vi "CTRnode.vi"(8 "error in":errorcluster) -> (0 "error out":errorcluster)   [LabVIEW 2024]
uses:
  Control/StreamCluster_TypeDef.ctl
  Control/streamIO_states.ctl
  <vilib>/Platform/TimedLoop/XDataNode/timing_clust.ctl
  <vilib>/Platform/TimedLoop/XDataNode/nitl_modes.ctl
  <vilib>/Platform/TimedLoop/XDataNode/wakeup.ctl
  Support/GlobalVars/StreamCluster.vi
  <vilib>/Platform/TimedLoop/TimeConversion.llb/rt-milliseconds-to-rel-time.vi
  <vilib>/Platform/TimedLoop/TimeConversion.llb/rt-milliseconds-to-timestamp.vi
  <vilib>/platform/TimedLoop/XDataNode/XDataNode.xnode
  <vilib>/Platform/TimedLoop/XDataNode/XDNodeRunTimeDep.lvlib
panel:
  out "element":dbl[][][](array[numeric])
  out "Manage Clock (ms)":cluster{"Period":i64, i64}(graph)
  out "Logging Clock (ms)":cluster{"Period":i64, i64}(graph)
  in  "stop":bool
  out "Streaming Clock (ms)":cluster{dbl, "Period":dbl}(graph)
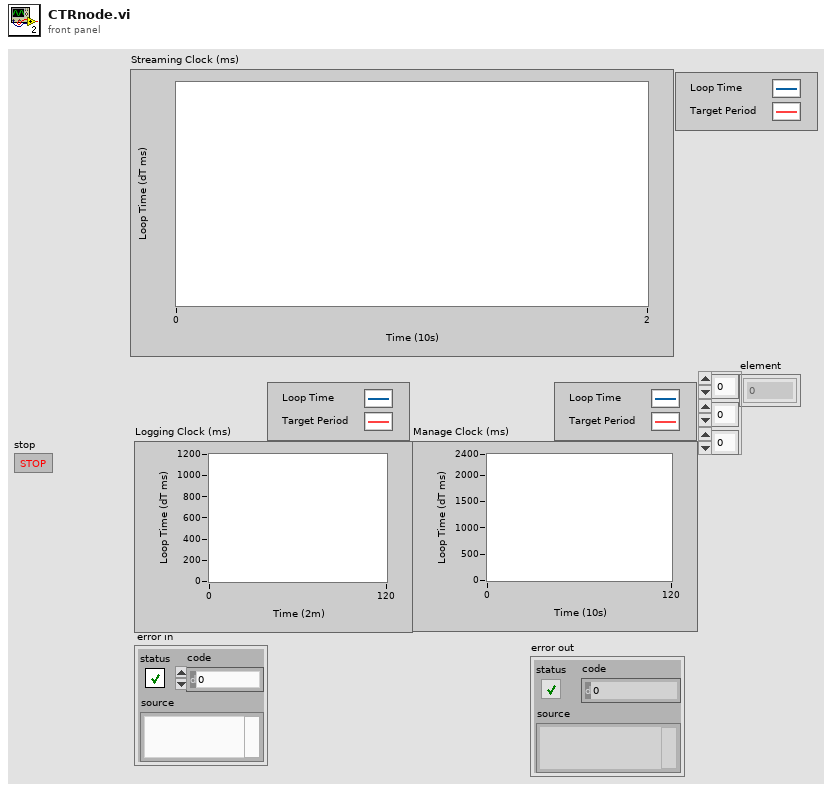
[diagram p1: front panel]
types:
  T1 = typedef "StreamCluster_TypeDef.ctl" = cluster{cluster{"stream state":T2, "TCP Remote Address":string, "TCP Connection ID":refnum<k5>, "DAQ Node":string, "DAQ Node ID":i32, "Writer Endpoint":refnum<k21>, "Reader Endpoint":refnum<k21>}[]}
  T2 = typedef "streamIO_states.ctl" = enum16{"Fault", "Initilize", "Stream", "Close"}
  T3 = typedef "XDNodeRunTimeDep.lvlib/timing_clust.ctl" = cluster{"Expected End [f-1]":u64, "Actual End [f-1]":u64, "Finished Late? [f-1]":bool, "Expected End [i-1]":u64, "Actual End [i-1]":u64, "Finished Late? [i-1]":bool, "Expected Start [i]":u64, "Actual Start [i]":u64, "Expected Start [f]":u64, "Actual Start [f]":u64, "Source Name":string, "Structure Name":string, "Period":i64, "Deadline":i64, "Offset":i64, "Start":i64, "Priority":i32, "Timeout":i32, "Mode":T4, "Wakeup Reason":T5, "Error":errorcluster, "Source Type":string, "Secondary Source Type":string, "Global End Time":u64, "Global Start Time":u64, "Frame Duration":u64, "Iteration Duration":u64, "Assigned CPU":i32, "I/O Scan Engine Mode":u32}
  T4 = typedef "XDNodeRunTimeDep.lvlib/nitl_modes.ctl" = enum32{"No Change", "Process missed periods, maintain original phase", "Discard missed periods, maintain original phase", "Process missed periods, ignore original phase", "Discard missed periods, ignore original phase"}
  T5 = typedef "XDNodeRunTimeDep.lvlib/wakeup.ctl" = enum32{"Normal", "Aborted", "Asynchronous wakeup", "Timing source error", "Timed loop error", "Timeout"}
  T6 = cluster{"stream state":T2, "TCP Remote Address":string, "TCP Connection ID":refnum<k5>, "DAQ Node":string, "DAQ Node ID":i32, "Writer Endpoint":refnum<k21>, "Reader Endpoint":refnum<k21>}[]
  T7 = cluster{"stream state":bool, "TCP Remote Address":bool, "TCP Connection ID":bool, "DAQ Node":bool, "DAQ Node ID":bool, "Writer Endpoint":bool, "Reader Endpoint":bool}
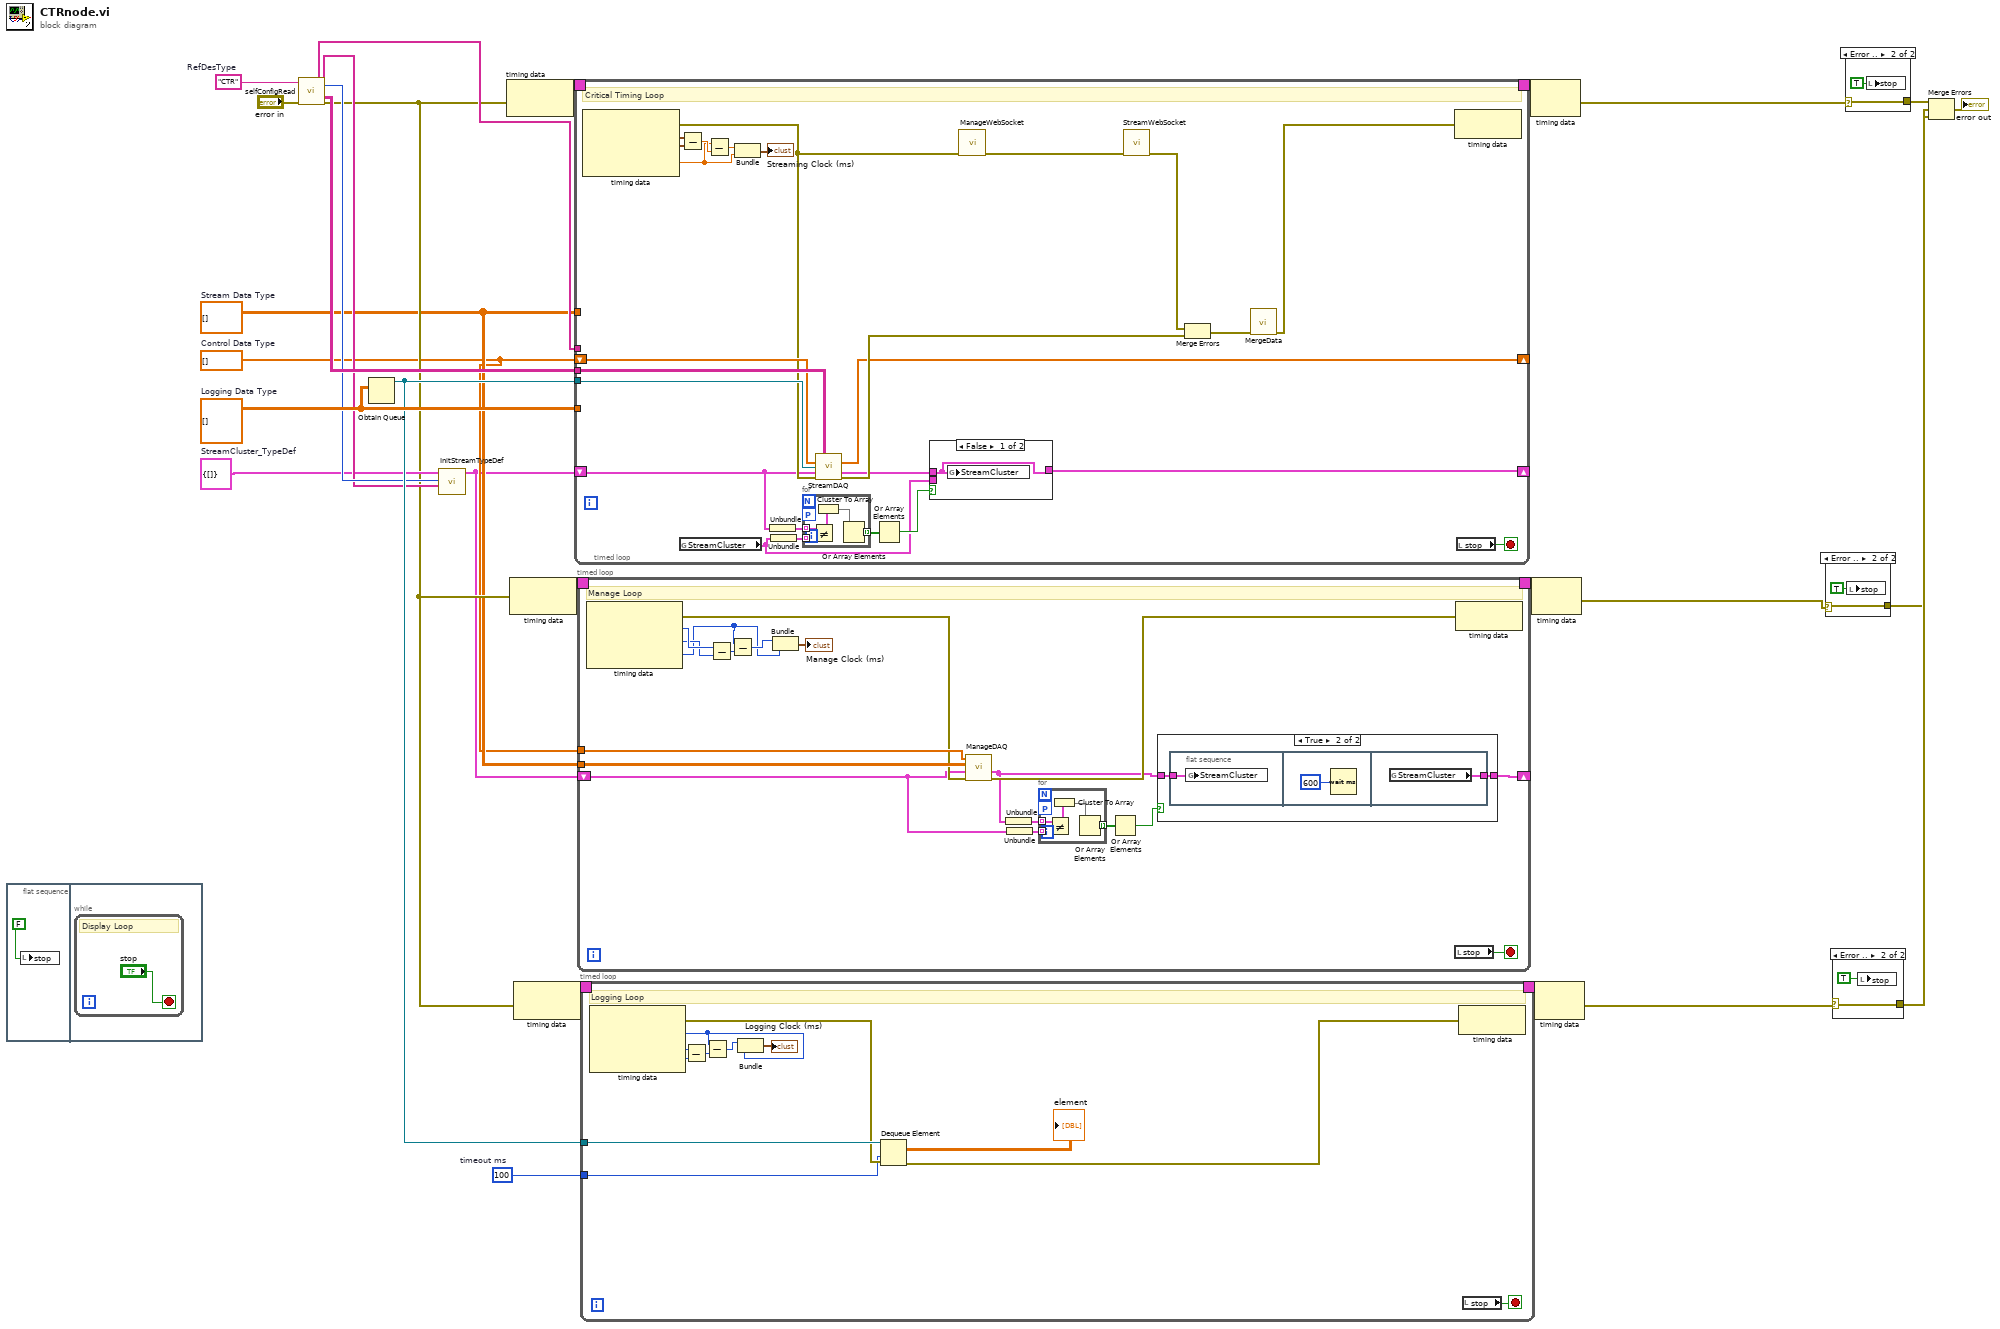
[diagram p0: block diagram]
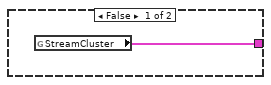
[diagram p3: hidden frame]
diagram:
  w9 = 100  # timeout ms
  w14 = T1 {[]}  # StreamCluster_TypeDef
  w4 = dbl[] []  # Control Data Type
  w20 = dbl[][][] []  # Logging Data Type
  w26 = "CTR"  # RefDesType
  w5 = dbl[][] []  # Stream Data Type
  n1 = flat-sequence {
    frame #0 {
      n2 = local write "stop"(FALSE ("stop")) -> ()
    }
    frame #1 {
      n3 = while {
        stop <- "stop" stop-if-true
        # "Display Loop"
      }
    }
  }
  n4 = call "selfConfigRead.vi"("RefDesType"=w26, "error in"="error in") -> ("Control refDes concat"=w19:string[], "DAQ Node Array"=w15:string[], "DAQ Node Count"=w16:i32, "Control refDes array"=w18:string[][], "error out"=w6:errorcluster)  [unwired: 11 in, 2 out]
  n5 = Obtain Queue(element data type=w20) -> (queue out=w17:refnum<queue>)  [unwired: 4 in, 2 out]
  n6 = call "InitStreamTypeDef.vi"("DAQ Node Array"=w15, "DAQ Node Count"=w16, "StreamCluster_TypeDef"=w14) -> ("StreamCluster_TypeDef"=w3:T1)  [unwired: 8 in]
  n7 = node-c288(w6) -> (w25:T3)
  n8 = node-c288(w6) -> (w8:T3)
  n9 = node-c288(w6) -> (w23:T3)
  n10 = timed-loop {
    timing: w25 -> [_]
    timing-out: [_] -> w24
    shift-right: [w30] -> _
    shift-left: w3 -> [w34]
    tunnel: w5 -> [_]
    tunnel: w20 -> [_]
    tunnel: w17 -> [w43]
    tunnel: w19 -> [_]
    tunnel: w18 -> [w42]
    shift-right: [w40] -> _
    shift-left: w4 -> [w39]
    stop <- w44 stop-if-true
    # "Critical Timing Loop"
    n11 = node-c288() -> (w38:errorcluster, w50:timestamp, w49:timestamp, w46:dbl)  [unwired: 1 in]
    n12 = global read "StreamCluster.vi" "StreamCluster"() -> (w31:T1)
    n13 = Subtract(x=w50, y=w49) -> (x-y=w48:dbl)
    n14 = Subtract(x=w46, y=w48) -> (x-y=w47:dbl)
    n15 = Bundle(w47, "Period"=w46) -> (→"Streaming Clock (ms)":cluster{dbl, "Period":dbl})  [unwired: 1 in]
    n16 = Unbundle(w34) -> (w37:T6)
    n17 = Unbundle(w31) -> (w36:T6)
    n18 = for {
      workers-P: _ -> [_]
      tunnel: w37 -> [w59] mode=indexing
      tunnel: w36 -> [w58] mode=indexing
      tunnel: [w55] -> w35 mode=indexing
      n19 = Not Equal?(x=w59, y=w58) -> (x != y?=w57:T7)
      n20 = Cluster To Array(cluster=w57) -> (array=w56:bool[])
      n21 = Or Array Elements(Boolean array=w56) -> (logical OR=w55:bool)
    }
    n22 = call "StreamDAQ.vi"("Control refDes array"=w42, "Control Data Type"=w39, "Logging Queue"=w43, "StreamCluster_TypeDef"=w34, "error in"=w38) -> ("Control Data Out"=w40:dbl[], "StreamCluster_TypeDef"=w32:T1, "error out"=w53:errorcluster)  [unwired: 8 in]
    n23 = Or Array Elements(Boolean array=w35) -> (logical OR=w33:bool)
    n24 = case shown="False" w33 {
      tunnel: w32 -> [w60 _]
      tunnel: w31 -> [_ w61]
      tunnel: [w60 w61] -> w30
      frame False {
        n25 = global write "StreamCluster.vi" "StreamCluster"(w60) -> ()
      }
      frame True {
      }
    }
    n26 = call "ManageWebSocket.vi"("error in"=w38) -> ("error out"=w51:errorcluster)  [unwired: 10 in]
    n27 = call "StreamWebSocket.vi"("error in"=w51) -> ("error out"=w52:errorcluster)  [unwired: 10 in]
    n28 = Merge Errors(w52, w53) -> (w54:errorcluster)
    n29 = call "MergeData.vi"("error in"=w54) -> ("error out"=w41:errorcluster)  [unwired: 10 in]
    n30 = node-c288(w41) -> ()  [unwired: 1 out]
    n31 = local read "stop"() -> (w44:bool)
  }
  n32 = timed-loop {
    timing: w8 -> [_]
    timing-out: [_] -> w7
    tunnel: w5 -> [w87]
    tunnel: w4 -> [w86]
    shift-right: [w83] -> _
    shift-left: w3 -> [w82]
    stop <- w88 stop-if-true
    # "Manage Loop"
    n33 = node-c288() -> (w85:errorcluster, w76:i64, w75:i64, w73:i64)  [unwired: 1 in]
    n34 = Subtract(x=w76, y=w75) -> (x-y=w90:i64)
    n35 = Subtract(x=w73, y=w90) -> (x-y=w74:i64)
    n36 = Bundle(w74, "Period"=w73) -> (→"Manage Clock (ms)":cluster{i64, "Period":i64})  [unwired: 1 in]
    n37 = call "ManageDAQ.vi"("error in"=w85, "StreamCluster_TypeDef"=w82, "Stream Data Type"=w87, "Control Data Type"=w86) -> ("error out"=w84:errorcluster, "StreamCluster_TypeDef"=w81:T1)  [unwired: 6 in]
    n38 = Unbundle(w81) -> (w80:T6)
    n39 = Unbundle(w82) -> (w79:T6)
    n40 = for {
      workers-P: _ -> [_]
      tunnel: w80 -> [w95] mode=indexing
      tunnel: w79 -> [w94] mode=indexing
      tunnel: [w91] -> w78 mode=indexing
      n41 = Not Equal?(x=w95, y=w94) -> (x != y?=w93:T7)
      n42 = Cluster To Array(cluster=w93) -> (array=w92:bool[])
      n43 = Or Array Elements(Boolean array=w92) -> (logical OR=w91:bool)
    }
    n44 = Or Array Elements(Boolean array=w78) -> (logical OR=w77:bool)
    n45 = case shown="True" w77 {
      tunnel: w81 -> [_ w98]
      tunnel: [w96 w97] -> w83
      frame False {
        n46 = global read "StreamCluster.vi" "StreamCluster"() -> (w96:T1)
      }
      frame True {
        n47 = flat-sequence {
          tunnel: w98 -> [w99]
          tunnel: [w101] -> w97
          frame #0 {
            n48 = global write "StreamCluster.vi" "StreamCluster"(w99) -> ()
          }
          frame #1 {
            n49 = Wait (ms)(milliseconds to wait=u32 600) -> ()  [unwired: 1 out]
          }
          frame #2 {
            n50 = global read "StreamCluster.vi" "StreamCluster"() -> (w101:T1)
          }
        }
      }
    }
    n51 = local read "stop"() -> (w88:bool)
    n52 = node-c288(w84) -> ()  [unwired: 1 out]
  }
  n53 = timed-loop {
    timing: w23 -> [_]
    timing-out: [_] -> w22
    tunnel: w17 -> [w116]
    tunnel: w9 -> [w113]
    stop <- w117 stop-if-true
    # "Logging Loop"
    n54 = node-c288() -> (w115:errorcluster, w110:i64, w119:i64, w120:i64)  [unwired: 1 in]
    n55 = Subtract(x=w119, y=w120) -> (x-y=w121:i64)
    n56 = Subtract(x=w110, y=w121) -> (x-y=w111:i64)
    n57 = Bundle(w111, "Period"=w110) -> (→"Logging Clock (ms)":cluster{i64, "Period":i64})  [unwired: 1 in]
    n58 = Dequeue Element(queue=w116, timeout in ms (-1)=w113, error in (no error)=w115) -> (element=→"element":dbl[][][], error out=w114:errorcluster)  [unwired: 2 out]
    n59 = node-c288(w114) -> ()  [unwired: 1 out]
    n60 = local read "stop"() -> (w117:bool)
  }
  n61 = node-c288(w24) -> (w13:errorcluster)
  n62 = node-c288(w7) -> (w1:errorcluster)
  n63 = node-c288(w22) -> (w11:errorcluster)
  n64 = case shown="Error .." w1 {
    selector: w1 -> [w130 w132]
    tunnel: [w130 w132] -> w2
    frame No Error {
    }
    frame Error {
      n65 = local write "stop"(TRUE ("stop")) -> ()
    }
  }
  n66 = case shown="Error .." w11 {
    selector: w11 -> [w133 w135]
    tunnel: [w133 w135] -> w10
    frame No Error {
    }
    frame Error {
      n67 = local write "stop"(TRUE ("stop")) -> ()
    }
  }
  n68 = case shown="Error .." w13 {
    selector: w13 -> [w136 w138]
    tunnel: [w136 w138] -> w12
    frame No Error {
    }
    frame Error {
      n69 = local write "stop"(TRUE ("stop")) -> ()
    }
  }
  n70 = Merge Errors(w12, w10, w2) -> (→"error out":errorcluster)
